vi "8.11.1.vi"() -> ()   [LabVIEW 2018]
panel:
  in  "데이터 전달":bool
  in  "송신 데이터":cluster{"이름":string, "토익 점수":dbl}
  out "소비 루프 반복":dbl
  out "수신 데이터":cluster{"이름":string, "토익 점수":dbl}
  out "생산 루프 반복":dbl
  in  "정지":bool
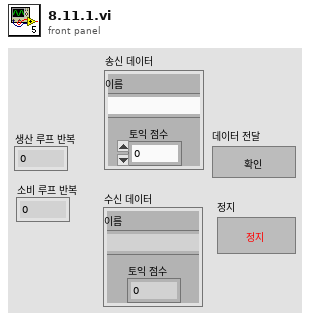
[diagram p1: front panel]
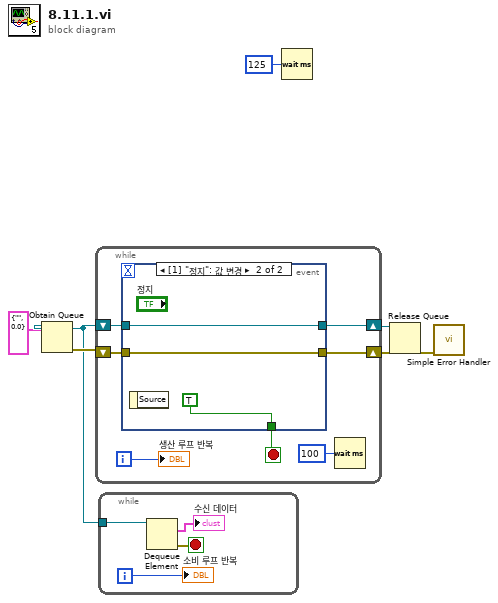
[diagram p0: block diagram]
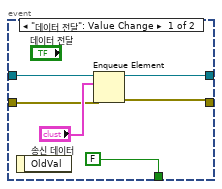
[diagram p2: hidden frame]
diagram:
  n1 = Obtain Queue(element data type=cluster{"이름":string, "토익 점수":dbl} {"이름"="", "토익 점수"=0.0} ("송신 데이터 2")) -> (queue out=w2:refnum<queue>, error out=w4:errorcluster)  [unwired: 4 in, 1 out]
  n2 = while {
    shift-right: [w11] -> w5
    shift-left: w2 -> [w12]
    shift-right: [w9] -> w3
    shift-left: w4 -> [w10]
    i -> [w14]
    stop <- w8 stop-if-true
    n3 = event shown="[1] \"정지\": 값 변경" {
      selector: _ -> [_ _]
      dyn-events: _ -> [_ _]
      timeout: _ -> [_ _]
      tunnel: w12 -> [w19 w22]
      tunnel: [w18 w22] -> w11
      tunnel: w10 -> [w17 w21]
      tunnel: [w16 w21] -> w9
      tunnel: [FALSE TRUE] -> w8
      event "데이터 전달": Value Change {
        n4 = event-data() -> ()  [unwired: 1 in, 1 out]
        n5 = Enqueue Element(queue=w19, element="송신 데이터", error in (no error)=w17) -> (queue out=w18:refnum<queue>, error out=w16:errorcluster)  [unwired: 1 in, 1 out]
      }
      event "정지": Value Change {
        n6 = event-data() -> ()  [unwired: 1 in, 1 out]
      }
    }
    n7 = Wait (ms)(milliseconds to wait=u32 100 ("대기 시간 (ms)")) -> ()  [unwired: 1 out]
    "생산 루프 반복" <- w14
  }
  n8 = while {
    tunnel: w2 -> [w25]
    i -> [w27]
    stop <- w26 stop-if-true
    n9 = Dequeue Element(queue=w25) -> (element=→"수신 데이터":cluster{"이름":string, "토익 점수":dbl}, error out=w26:errorcluster)  [unwired: 2 in, 2 out]
    "소비 루프 반복" <- w27
  }
  n10 = Wait (ms)(milliseconds to wait=u32 125 ("대기 시간 (ms)")) -> ()  [unwired: 1 out]
  n11 = Release Queue(queue=w5, error in (no error)=w3) -> (error out=w6:errorcluster)  [unwired: 1 in, 2 out]
  n12 = call <vilib>:"Simple Error Handler.vi"("error in (no error)"=w6) -> ()  [unwired: 4 in, 5 out]
